vi "sendAckToClient.vi"(8 "error in (no error)":errorcluster, 9 "cmdStatus":string(combo)="ack", 10 "Ack":string="command received", 11 "tcpServer in":refnum<class "TcpServer.lvclass">) -> (0 "error out":errorcluster, 3 "tcpServer out":refnum<class "TcpServer.lvclass">)   [LabVIEW 2018, in "TcpServer.lvclass"]
doc: "Send the Ack to the Tcp Client."
uses:
  TcpServer.lvclass
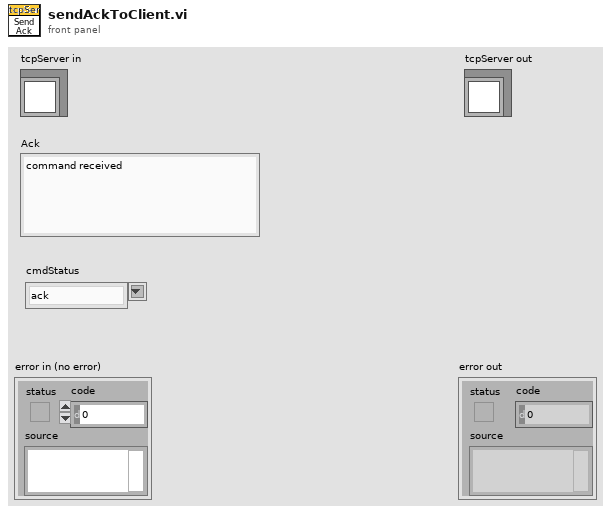
[diagram p1: front panel]
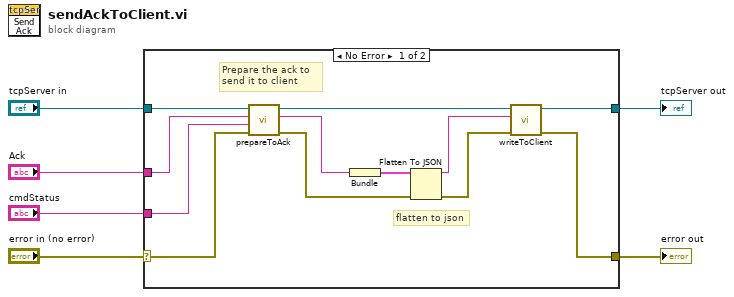
[diagram p0: block diagram]
diagram:
  n1 = case shown="No Error" "error in (no error)" {
    selector: "error in (no error)" -> [w9 w20]
    tunnel: [w17 w20] -> w5
    tunnel: [w18 w19] -> w3
    tunnel: "tcpServer in" -> [w13 w19]
    tunnel: "Ack" -> [w11 _]
    tunnel: "cmdStatus" -> [w7 _]
    frame No Error {
      # "Prepare the ack to\nsend it to client"
      # "flatten to json"
      n2 = call "prepareToAck.vi"("error in (no error)"=w9, "cmdStatus"=w7, "command"=w11, "TcpServer in"=w13) -> ("error out"=w8:errorcluster, "JSON string"=w10:string, "TcpServer out"=w12:refnum<class "TcpServer.lvclass">)  [unwired: 5 in]
      n3 = Bundle("JSON string"=w10) -> (w16:cluster{"JSON string":string})  [unwired: 1 in]
      n4 = Flatten To JSON(anything=w16, error in (no error)=w8) -> (JSON string=w15:string, 11:w14:errorcluster)  [unwired: 1 in]
      n5 = call "writeToClient.vi"("error in (no error)"=w14, "packet"=w15, "tcpServer in"=w12) -> ("error out"=w17:errorcluster, "tcpServer out"=w18:refnum<class "TcpServer.lvclass">)  [unwired: 7 in]
    }
    frame Error {
    }
  }
  "error out" <- w5
  "tcpServer out" <- w3
